vi "Fetch Waveforms.vi"(8 "error in":errorcluster, 11 "object in":refnum<class "Scope PXI CFG.lvclass">) -> (0 "error out":errorcluster, 2 "Last Waveforms":map{u8, waveform(dbl)}(c390), 3 "object out":refnum<class "Scope PXI CFG.lvclass">)   [LabVIEW 2023, in "Scope.lvlib" / "Scope PXI.lvlib" / "Scope PXI CFG.lvclass"]
uses:
  Scope PXI CFG.lvclass
  Scope PXI CFG.lvclass/Scope PXI CFG.ctl
  Configuration Base/Configuration Base.lvclass
  8d36052f-398f-4416-96a9-5ca09e3acc97.vi
  ce682fe7-8147-45a0-826f-6225c648e612.vi
  02167e95-eb1b-459e-9628-7c497ad36d0b.vi
  <instrlib>/niScope/Controls/niScope timestamp type.ctl
  d9bd0854-c9e2-4517-b292-7db69c37fda0.vi
  <instrlib>/niScope/Acquire/Fetch/niScope Fetch WDT.vi
  <vilib>/ErrorRing/Error Ring.xnode
  <vilib>/Utility/error.llb/Error Cluster From Error Code.vi
  D:/git/HAL/Configuration Base/Configuration Base.lvclass
  D:/git/HAL/Interfaces/IConfigure/IConfigure.lvclass
  D:/git/HAL/Scope PXI/Scope PXI CFG/Scope PXI CFG.lvclass
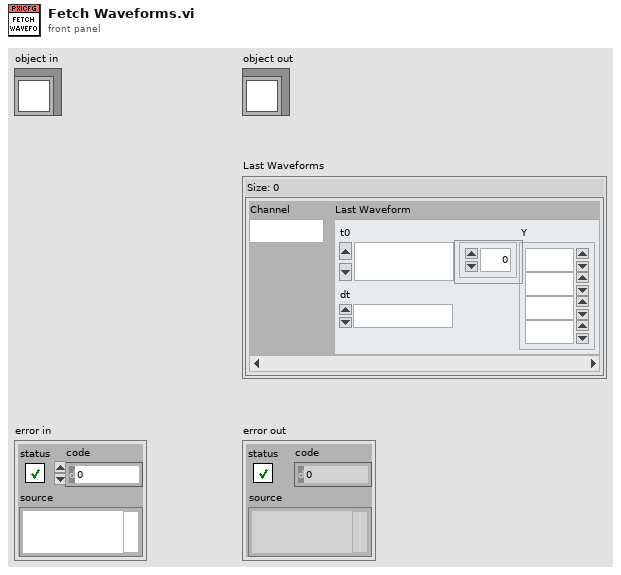
[diagram p1: front panel]
types:
  T1 = typedef "niScope timestamp type.ctl" = i32
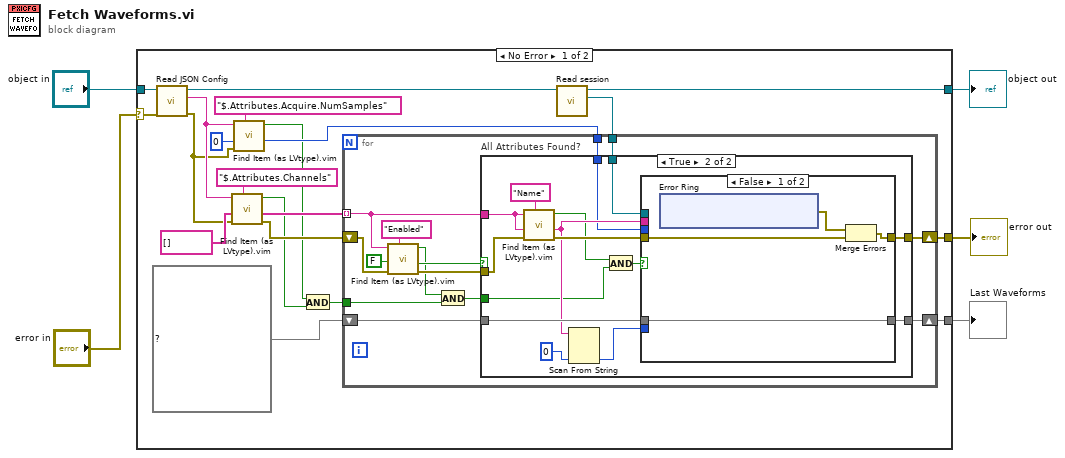
[diagram p0: block diagram]
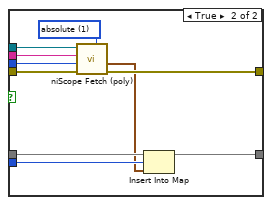
[diagram p3: hidden frame]
diagram:
  n1 = case shown="No Error" "error in" {
    selector: "error in" -> [w14 w77]
    tunnel: [w25 w76] -> w5
    tunnel: "object in" -> [w24 w76]
    tunnel: [w16 _] -> w3
    tunnel: [w15 w77] -> w2
    frame No Error {
      n2 = call "Read JSON Config.vi"("error in"=w14, "object in"=w24) -> ("error out"=w11:errorcluster, "<JSON>Config"=w13:string, "object out"=w23:refnum<class "Scope PXI CFG.lvclass">)  [unwired: 7 in]
      n3 = call "Find Item (as LVtype).vim"("$Path or Item Name"="$.Attributes.Channels", "error in (no error)"=w11, "Data Type and Default Value"=string[] [], "JSON"=w13) -> ("error out"=w19:errorcluster, "Data"=w20:string[], "Found"=w7:bool)  [unwired: 4 in, 1 out]
      n4 = call "Find Item (as LVtype).vim"("$Path or Item Name"="$.Attributes.Acquire.NumSamples", "error in (no error)"=w11, "Data Type and Default Value"=0, "JSON"=w13) -> ("Data"=w9:i32, "Found"=w8:bool)  [unwired: 4 in, 2 out]
      n5 = And(x=w8, y=w7) -> (x .and. y?=w6:bool)
      n6 = call "Read session.vi"("Scope PXI CFG in"=w23) -> ("session"=w18:refnum<k15>, "Scope PXI CFG out"=w25:refnum<class "Scope PXI CFG.lvclass">)  [unwired: 8 in, 1 out]
      n7 = for {
        tunnel: w20 -> [w34] mode=indexing
        tunnel: w18 -> [w33]
        shift-right: [w32] -> w15
        shift-left: w19 -> [w39]
        shift-right: [w30] -> w16
        shift-left: map{u8, waveform(dbl)} {} ("Last Waveforms") -> [w31]
        tunnel: w9 -> [w29]
        tunnel: w6 -> [w26]
        n8 = call "Find Item (as LVtype).vim"("$Path or Item Name"="Enabled", "error in (no error)"=w39, "Data Type and Default Value"=FALSE, "JSON"=w34) -> ("error out"=w36:errorcluster, "Data"=w35:bool, "Found"=w28:bool)  [unwired: 4 in, 1 out]
        n9 = And(x=w28, y=w26) -> (x .and. y?=w27:bool)
        n10 = case "All Attributes Found?" shown="True" w35 {
          tunnel: w36 -> [w40 w56]
          tunnel: w34 -> [_ w49]
          tunnel: w33 -> [_ w54]
          tunnel: [w40 w52] -> w32
          tunnel: w31 -> [w41 w51]
          tunnel: [w41 w50] -> w30
          tunnel: w29 -> [_ w45]
          tunnel: w27 -> [_ w42]
          frame False {
          }
          frame True {
            n11 = call "Find Item (as LVtype).vim"("$Path or Item Name"="Name", "error in (no error)"=w56, "Data Type and Default Value"=w49, "JSON"=w49) -> ("error out"=w53:errorcluster, "Data"=w48:string, "Found"=w43:bool)  [unwired: 4 in, 1 out]
            n12 = Scan From String(input string=w48, default 1=u8 0 ("key")) -> (output 1=w46:u8)  [unwired: 3 in, 3 out]
            n13 = And(x=w43, y=w42) -> (x .and. y?=w44:bool)
            n14 = case shown="False" w44 {
              tunnel: w54 -> [_ w75]
              tunnel: w53 -> [w60 w74]
              tunnel: [w58 w73] -> w52
              tunnel: w51 -> [w59 w72]
              tunnel: [w59 w71] -> w50
              tunnel: w48 -> [_ w70]
              tunnel: w46 -> [_ w69]
              tunnel: w45 -> [_ w66]
              frame False {
                n15 = xnode "Error Ring"() -> ("error out"=w57:errorcluster)
                n16 = Merge Errors(w57, w60) -> (w58:errorcluster)
              }
              frame True {
                w67 = T1 1 items=["relative", "absolute"] ("timestamp Type")
                n17 = call-poly <instrlib>:"niScope Fetch (poly).vi"("timestamp Type"=w67, "error in"=w74, "numSamples"=w66, "channels"=w70, "instrument handle"=w75) -> ("error out"=w73:errorcluster, "wfm"=w68:waveform(dbl))  [unwired: 3 in, 2 out]
                n18 = Insert Into Map(map in=w72, key=w69, value=w68) -> (map out=w71:map{u8, waveform(dbl)})  [unwired: 2 out]
              }
            }
          }
        }
      }
    }
    frame Error {
    }
  }
  "error out" <- w2
  "object out" <- w5
  "Last Waveforms" <- w3
